vi "Get Original FIFO Channel Name.vi"(11 "Channel Name":string) -> (3 "Original Channel Name":string)   [LabVIEW 2021, in "CIFChannelMng.lvclass"]
uses:
  CIFChannelMng.lvclass
  CIFChannelMng.lvclass/CIFChannelMng.ctl
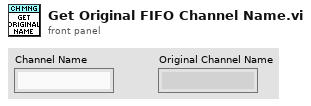
[diagram p1: front panel]
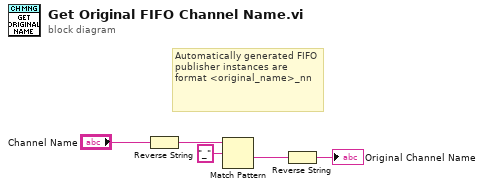
[diagram p0: block diagram]
diagram:
  # "Automatically generated FIFO publisher instances are format <original_name>_nn"
  n1 = Reverse String(1:"Channel Name") -> (0:w4:string)
  n2 = Match Pattern(string=w4, regular expression="_") -> (after substring=w2:string)  [unwired: 1 in, 3 out]
  n3 = Reverse String(1:w2) -> (0:→"Original Channel Name":string)
